vi "tEST.vi"(8 "error in (no error)":errorcluster, 11 "SQL Saver in":refnum<class "SQL Saver.lvclass">) -> (0 "error out":errorcluster, 3 "SQL Saver out":refnum<class "SQL Saver.lvclass">)   [LabVIEW 2015, in "Data Saving.lvlib" / "SQL Saver.lvclass"]
uses:
  SQL Saver.lvclass
  <vilib>/addons/database/Connection.llb/DB Tools Open Connec (String).vi
  <vilib>/addons/database/NI_Database_API.lvlib
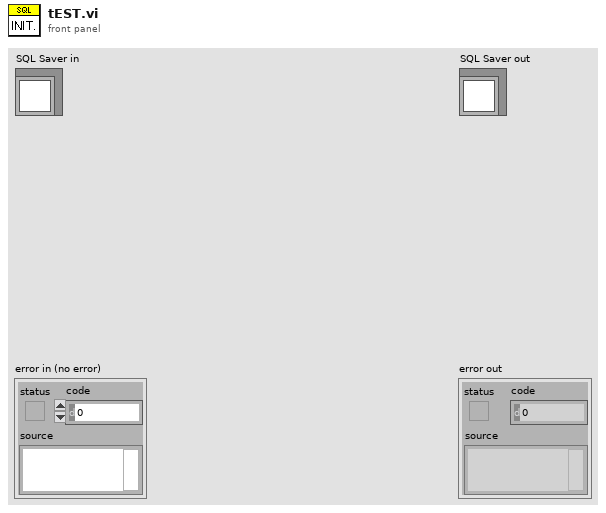
[diagram p1: front panel]
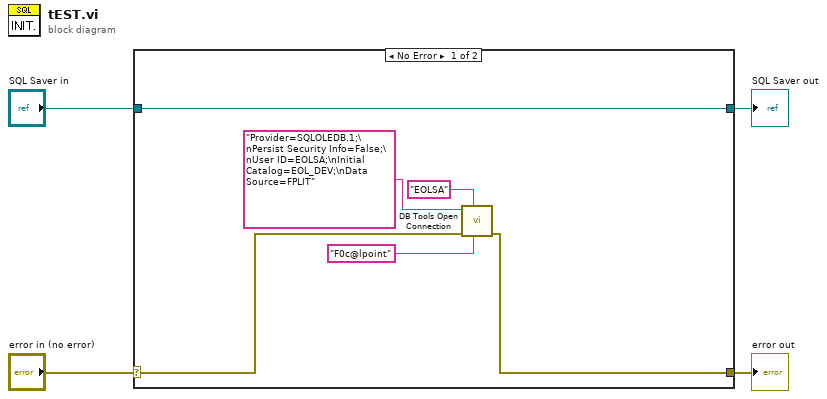
[diagram p0: block diagram]
diagram:
  n1 = case shown="No Error" "error in (no error)" {
    selector: "error in (no error)" -> [w6 w12]
    tunnel: [w5 w12] -> w3
    tunnel: [w10 w11] -> w1
    tunnel: "SQL Saver in" -> [w10 w11]
    frame No Error {
      n2 = call-poly <vilib>:"DB Tools Open Connection.vi"("password"="F0c@lpoint", "userID"="EOLSA", "error in (no error)"=w6, "connection information"="Provider=SQLOLEDB.1;\nPersist Security Info=False;\nUser ID=EOLSA;\nInitial Catalog=EOL_DEV;\nData Source=FPLIT" ("ConnectionString")) -> ("error out"=w5:errorcluster)  [unwired: 4 in, 1 out]
    }
    frame Error {
    }
  }
  "error out" <- w3
  "SQL Saver out" <- w1
